vi "Save Transport DAT File.vi"(8 "error in (no error)":errorcluster, 10 "Data (Row)":dbl[](array[numeric]), 11 "Control Experiment":refnum<class "Control Experiment.lvclass">) -> (0 "error out":errorcluster, 3 "Control Experiment out":refnum<class "Control Experiment.lvclass">)   [LabVIEW 2016, in "Control Experiment.lvclass"]
uses:
  Control Experiment.lvclass
  <userlib>/LevyLab/LV to ITX/Data/Data.lvclass
  <userlib>/LevyLab/LV to ITX/Data/Typedefs/File Type--enum.ctl
  <userlib>/LevyLab/LV to ITX/Data/Typedefs/Dictionary--cluster.ctl
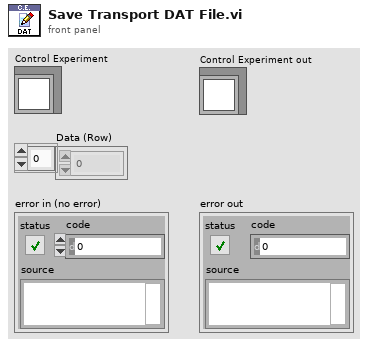
[diagram p1: front panel]
types:
  T1 = typedef "Data.lvclass/File Type--enum.ctl" = enum16{"DAT", "ITX", "TDMS", "VI"}
  T2 = typedef "Data.lvclass/Dictionary--cluster.ctl" = cluster{"key":string, "value":variant}
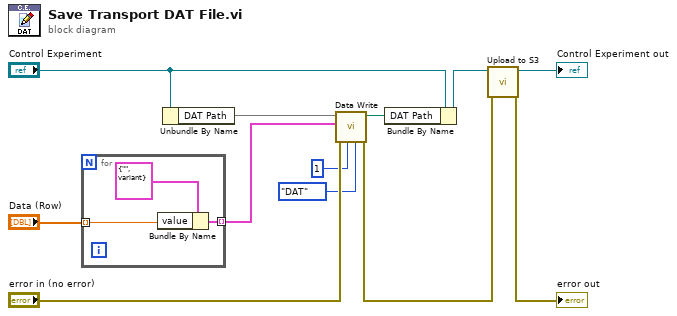
[diagram p0: block diagram]
diagram:
  n1 = for {
    tunnel: "Data (Row)" -> [w14] mode=indexing
    tunnel: [w13] -> w7 mode=indexing
    n2 = Bundle By Name(cluster=T2 {"key"="", "value"=variant} ("key-value"), "value"=w14) -> (w13:T2)
  }
  n3 = Unbundle By Name("Control Experiment") -> ("DAT Path"=w12)
  n4 = call <userlib>:"Data Write.vi"("File Type"=File_Type--enum."DAT", "Append Index"=1, "error in (no error)"="error in (no error)", "Data (Dictionary)"=w7, "path"=w12) -> ("error out"=w2:errorcluster, "path out"=w6:path)  [unwired: 5 in]
  n5 = Bundle By Name(cluster="Control Experiment", "DAT Path"=w6) -> (w4:refnum<class "Control Experiment.lvclass">)
  n6 = call "Upload to S3.vi"("error in (no error)"=w2, "Control Experiment"=w4) -> ("error out"=→"error out":errorcluster, "Control Experiment out"=→"Control Experiment out":refnum<class "Control Experiment.lvclass">)  [unwired: 8 in]
